vi "VisionExecute.vi"(8 "error in (no error)":errorcluster, 9 "Vision enabled?":bool, 11 "Vision in":refnum<class "Vision.lvclass">) -> (0 "error out":errorcluster, 1 "Vision Finished?":bool, 3 "Vision out":refnum<class "Vision.lvclass">)   [LabVIEW 2018, in "Vision.lvclass"]
uses:
  Vision.lvclass
  Vision.lvclass/Vision.ctl
  <vilib>/Rock Robotics/WPI/ThirdParty/Phoenix-LabVIEW/Motor Controller/Controls/CTRE_Phoenix_MotorControl_ControlMode.ctl
  69fdfca0-1e75-464e-9cf5-3e9e15e61420.vi
  <vilib>/addons/control/pid/pid.llb/PID (DBL).vi
  <vilib>/addons/control/pid/NI_PID_pid.lvlib
panel:
  out "Waveform Chart":dynamicdata(graph)
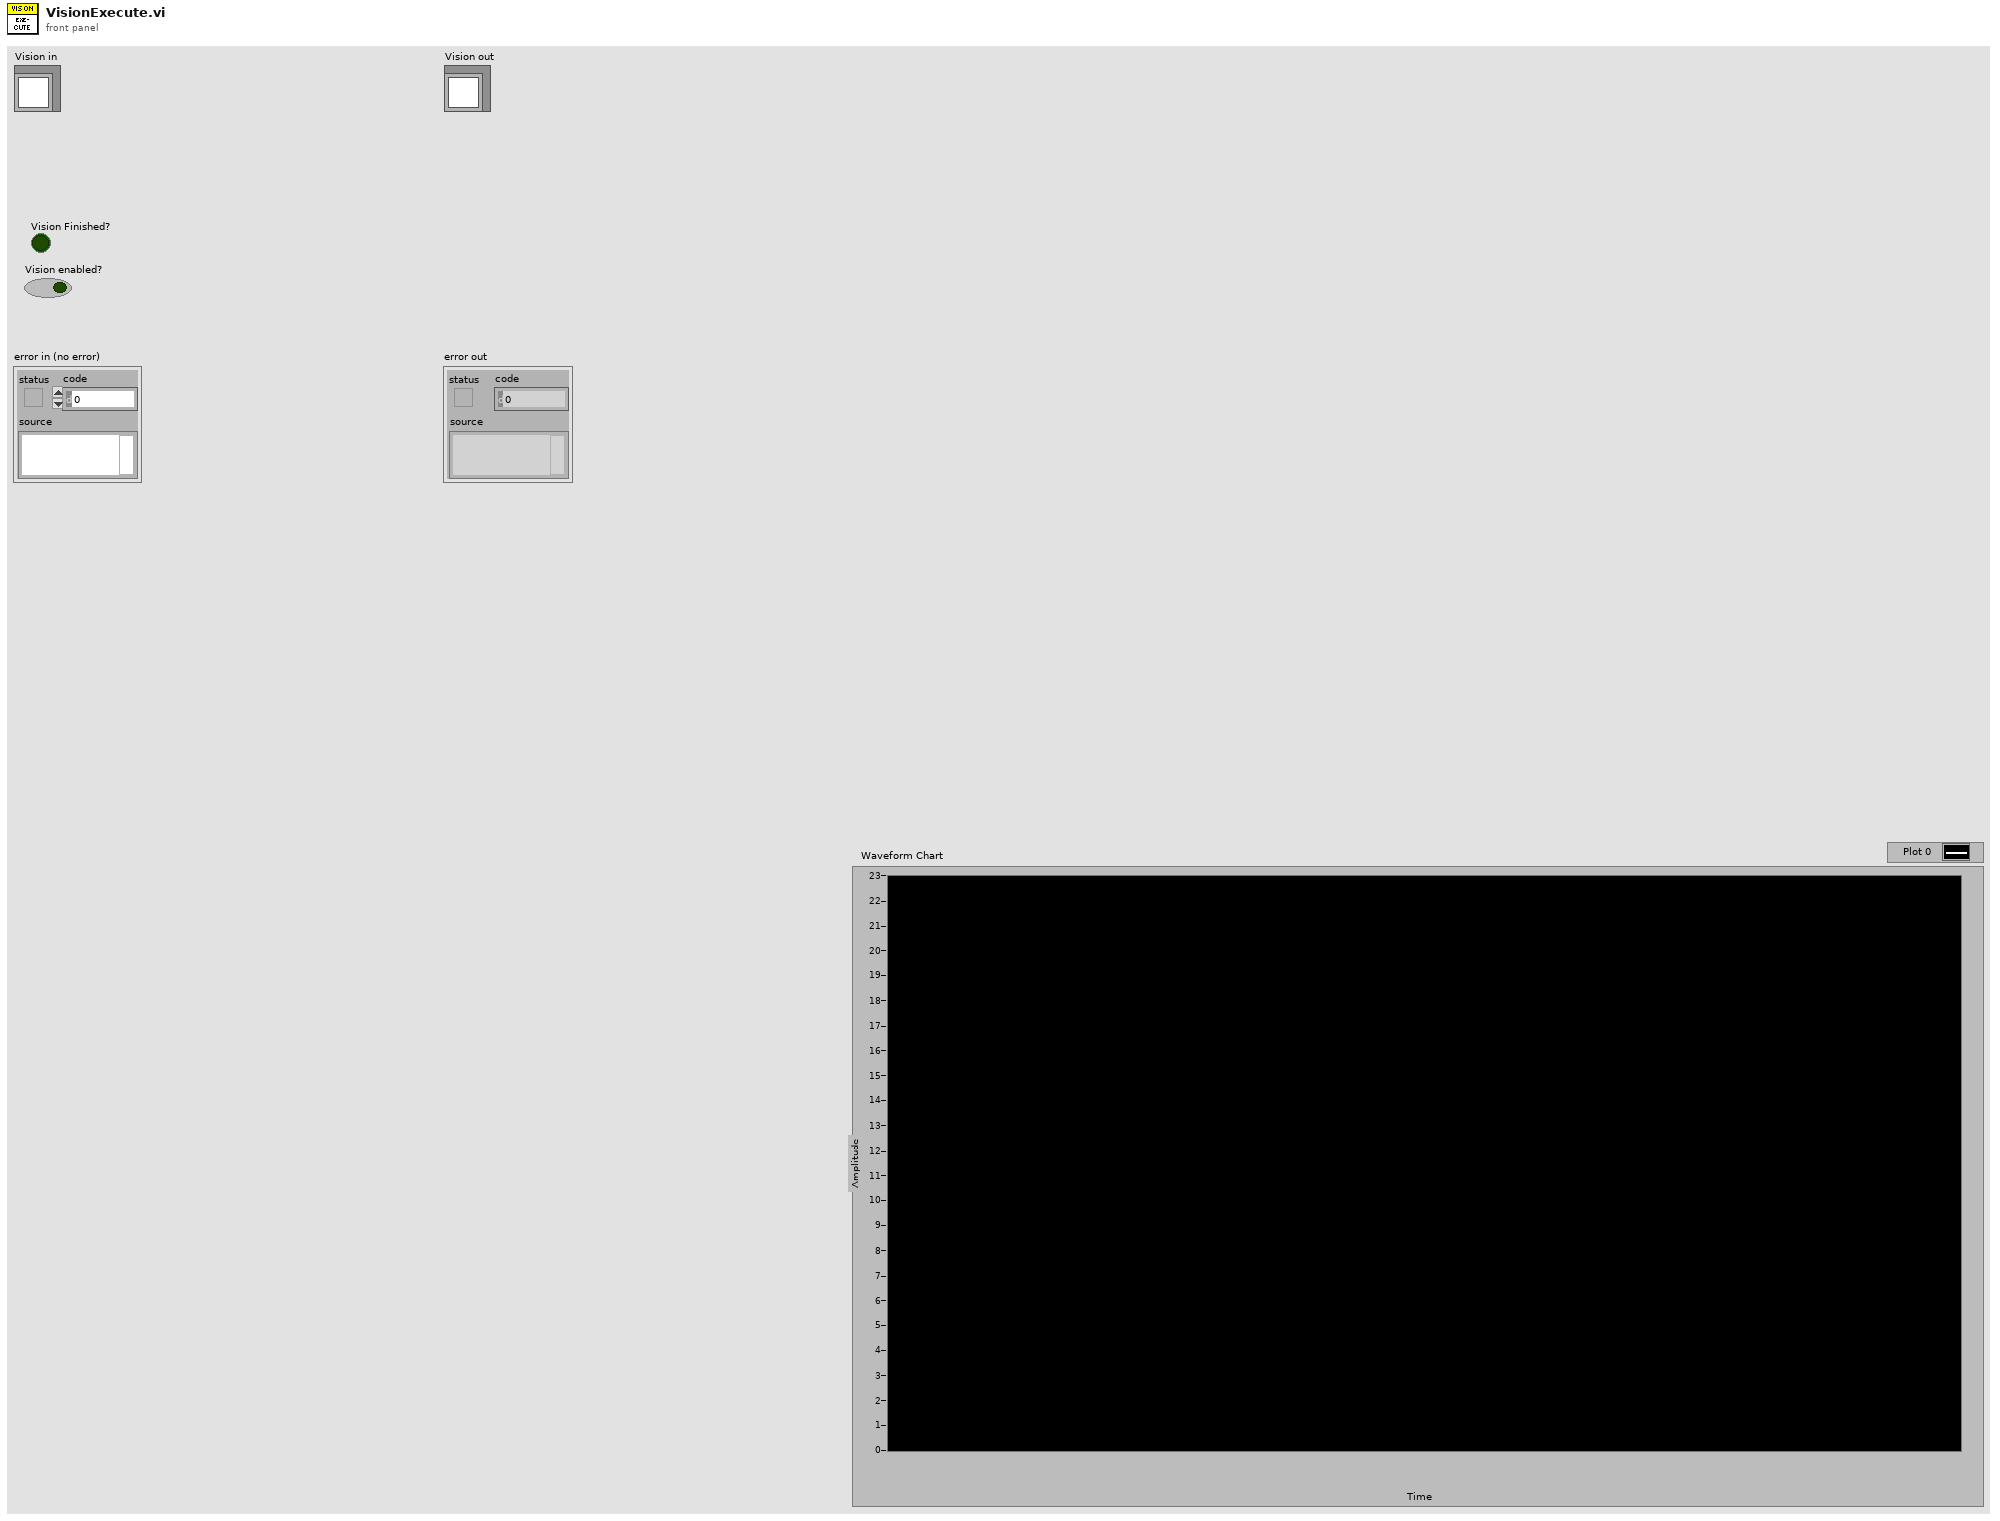
[diagram p1: front panel]
types:
  T1 = typedef "CTRE_Phoenix_MotorControl_ControlMode.ctl" = u16
  T2 = cluster{"proportional gain (Kc)":dbl, "integral time (Ti, min)":dbl, "derivative time (Td, min)":dbl}
  T3 = typedef "WPI_MotorControlDeviceRef.ctl" = cluster{"DeviceStatus":errorcluster, "Type":T4, "PWM":cluster{"PWM Channel":T5, "DeadBand":T6}, "CAN":cluster{"Device Number":u8, "SetOutput VI Ref":variant, "GetOutput VI Ref":variant, "Enable VI Ref":variant, "Disable VI Ref":variant, "Data":variant}, "Invert":bool, "DIO PWM":cluster{"PWM \"Enable\" Channel":T5, "DIOChannel":T7, "PWM Rate":dbl}}
  T4 = typedef "WPI_MotorControlType.ctl" = enum16{"PWM", "CAN", "DIO PWM"}
  T5 = typedef "FPGA_DIOPWMChannel.ctl" = enum8{"PWM 0", "PWM 1", "PWM 2", "PWM 3", "PWM 4", "PWM 5", "PWM 6", "PWM 7", "PWM 8", "PWM 9", "PWM MXP 0", "PWM MXP 1", "PWM MXP 2", "PWM MXP 3", "PWM MXP 4", "PWM MXP 5", "PWM MXP 6", "PWM MXP 7", "PWM MXP 8", "PWM MXP 9", "Invalid"}
  T6 = typedef "WPI_PWMDeadband.ctl" = cluster{"Name":string, "maxPositivePwm":i32, "minPositivePwm":i32, "centerPwm":i32, "maxNegativePwm":i32, "minNegativePwm":i32, "angularRange":u16}
  T7 = typedef "FPGA_DIOChannel.ctl" = enum8{"DIO 0", "DIO 1", "DIO 2", "DIO 3", "DIO 4", "DIO 5", "DIO 6", "DIO 7", "DIO 8", "DIO 9", "DIO MXP 0", "DIO MXP 1", "DIO MXP 2", "DIO MXP 3", "DIO MXP 4", "DIO MXP 5", "DIO MXP 6", "DIO MXP 7", "DIO MXP 8", "DIO MXP 9", "DIO MXP 10", "DIO MXP 11", "DIO MXP 12", "DIO MXP 13", "DIO MXP 14", "DIO MXP 15", "SPI Port CS1", "SPI Port CS2", "SPI Port CS3", "SPI Port MISO", "SPI Port MOSI", "Invalid"}
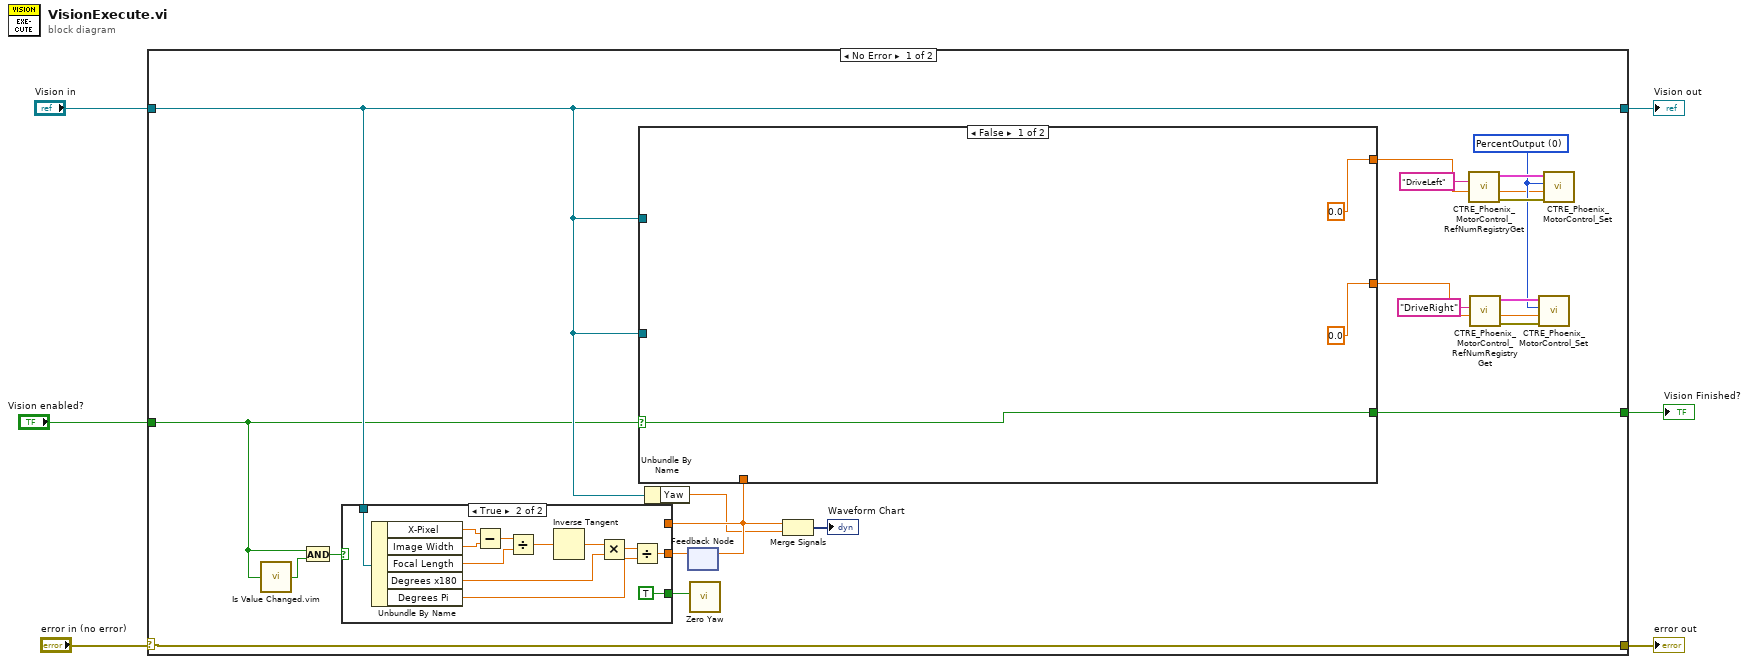
[diagram p0: block diagram]
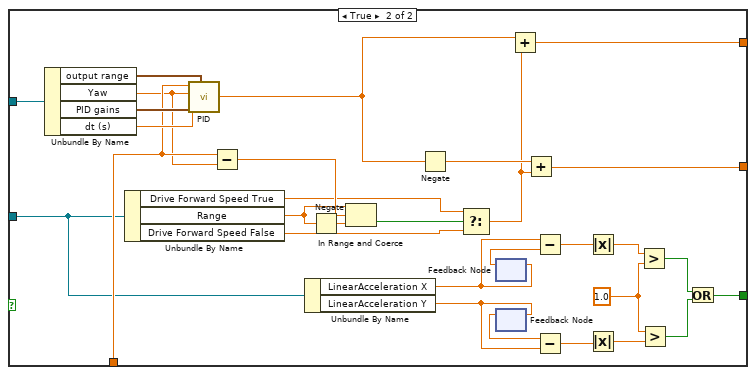
[diagram p2: hidden frame]
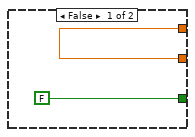
[diagram p3: hidden frame]
diagram:
  n1 = case shown="No Error" "error in (no error)" {
    selector: "error in (no error)" -> [w7 w76]
    tunnel: [w7 w76] -> w5
    tunnel: [w14 w75] -> w3
    tunnel: "Vision in" -> [w14 w75]
    tunnel: "Vision enabled?" -> [w9 w74]
    tunnel: [w8 w74] -> w1
    frame No Error {
      w18 = T1 0 items=["PercentOutput"=0, "Position"=1, "Velocity"=2, "Current"=3, "Follower"=5, "MotionProfile"=6, "MotionMagic"=7, "MotionProfileArc"=10, "Disabled"=15] ("Control Mode")
      n2 = call "Is Value Changed.vim"("value"=w9) -> ("changed or first call?"=w23:bool)
      n3 = And(x=w9, y=w23) -> (x .and. y?=w26:bool)
      n4 = Unbundle By Name(w14) -> ("Yaw"=w15:dbl)
      n5 = feedback #1() -> (w16:dbl)  [unwired: 1 in]
      n6 = case shown="True" w26 {
        tunnel: [FALSE TRUE] -> w25
        tunnel: [w60 w68] -> w24
        tunnel: w16 -> [w60 _]
        tunnel: w14 -> [_ w67]
        frame False {
        }
        frame True {
          n7 = Unbundle By Name(w67) -> ("X-Pixel"=w66:dbl, "Image Width"=w65:dbl, "Focal Length"=w64:dbl, "Degrees x180"=w63:dbl, "Degrees Pi"=w62:dbl)
          n8 = Subtract(x=w66, y=w65) -> (x-y=w72:dbl)
          n9 = Divide(x=w72, y=w64) -> (x/y=w71:dbl)
          n10 = Inverse Tangent(1:w71) -> (0:w70:dbl)
          n11 = Multiply(x=w70, y=w63) -> (x*y=w69:dbl)
          n12 = Divide(x=w69, y=w62) -> (x/y=w68:dbl)
        }
      }
      n13 = case shown="False" w9 {
        selector: w9 -> [w27 _]
        tunnel: [0.0 w55] -> w10
        tunnel: [0.0 w54] -> w11
        tunnel: w14 -> [_ w53]
        tunnel: w14 -> [_ w42]
        tunnel: w16 -> [_ w44]
        tunnel: [w27 w30] -> w8
        frame False {
        }
        frame True {
          w35 = 1.0
          n14 = Unbundle By Name(w53) -> ("output range"=w52:cluster{"output high":dbl, "output low":dbl}, "Yaw"=w43:dbl, "PID gains"=w51:T2, "dt (s)"=w50:dbl)
          n15 = Unbundle By Name(w42) -> ("Drive Forward Speed True"=w47:dbl, "Range"=w46:dbl, "Drive Forward Speed False"=w45:dbl)
          n16 = call-poly <vilib>:"PID.vi"("output range"=w52, "dt (s)"=w50, "PID gains"=w51, "process variable"=w43, "setpoint"=w44) -> ("output"=w58:dbl)  [unwired: 5 in, 1 out]
          n17 = Subtract(x=w44, y=w43) -> (x-y=w48:dbl)
          n18 = Unbundle By Name(w42) -> ("LinearAcceleration X"=w39:dbl, "LinearAcceleration Y"=w38:dbl)
          n19 = Negate(x=w46) -> (-x=w49:dbl)
          n20 = In Range and Coerce(upper limit=w46, x=w48, lower limit=w49) -> (In Range?=w57:bool)  [unwired: 1 out]
          n21 = Negate(x=w58) -> (-x=w59:dbl)
          n22 = Select(t=w47, s=w57, f=w45) -> (s? t:f=w56:dbl)
          n23 = feedback #2() -> (w41:dbl)  [unwired: 1 in]
          n24 = feedback-in #2(w39) -> ()
          n25 = feedback #3() -> (w40:dbl)  [unwired: 1 in]
          n26 = feedback-in #3(w38) -> ()
          n27 = Add(x=w58, y=w56) -> (x+y=w54:dbl)
          n28 = Add(x=w59, y=w56) -> (x+y=w55:dbl)
          n29 = Subtract(x=w39, y=w41) -> (x-y=w31:dbl)
          n30 = Subtract(x=w40, y=w38) -> (x-y=w32:dbl)
          n31 = Absolute Value(x=w31) -> (abs(x)=w36:dbl)
          n32 = Absolute Value(x=w32) -> (abs(x)=w37:dbl)
          n33 = Greater?(x=w36, y=w35) -> (0:w33:bool)
          n34 = Greater?(x=w35, y=w37) -> (0:w34:bool)
          n35 = Or(x=w33, y=w34) -> (x .or. y?=w30:bool)
        }
      }
      n36 = feedback-in #1(w24) -> ()
      n37 = call <vilib>:"Zero Yaw.vi"("Zero"=w25) -> ()  [unwired: 11 in]
      n38 = Merge Signals(w16, w15) -> (→"Waveform Chart":dynamicdata)
      n39 = call <vilib>:"CTRE_Phoenix_MotorControl_RefNumRegistryGet.vi"("refnum name"="DriveLeft") -> ("error out"=w20:errorcluster, "PhoenixMotorControlDevRef"=w19:T3)  [unwired: 9 in]
      n40 = call <vilib>:"CTRE_Phoenix_MotorControl_RefNumRegistryGet.vi"("refnum name"="DriveRight") -> ("error out"=w21:errorcluster, "PhoenixMotorControlDevRef"=w22:T3)  [unwired: 9 in]
      n41 = call <vilib>:"CTRE_Phoenix_MotorControl_Set.vi"("error in (no error)"=w21, "Output"=w10, "Control Mode"=w18, "PhoenixMotorControlDevRef"=w22) -> ()  [unwired: 6 in, 2 out]
      n42 = call <vilib>:"CTRE_Phoenix_MotorControl_Set.vi"("error in (no error)"=w20, "Output"=w11, "Control Mode"=w18, "PhoenixMotorControlDevRef"=w19) -> ()  [unwired: 6 in, 2 out]
    }
    frame Error {
    }
  }
  "error out" <- w5
  "Vision out" <- w3
  "Vision Finished?" <- w1
